vi "SFC_Get SOInfo.vi"(7 "UserNo":string, 8 "error in (no error)":errorcluster caption="错误输入（无错误）", 9 "Model":string, 10 "SalesOrder":string, 11 "Traceability 引用句柄":refnum<k24>) -> (0 "error out":errorcluster caption="错误输出", 2 ".NET:System.Data.DataSet":T1={"CaseSensitive"=FALSE, "Container"=refnum, "DataSetName"="", "DefaultViewManager"=refnum, "DesignMode"=FALSE, "EnforceConstraints"=FALSE, "ExtendedProperties"=refnum, "HasErrors"=FALSE, "IsInitialized"=FALSE, "Locale"=refnum, "Namespace"="", "Prefix"="", "Relations"=refnum, "RemotingFormat"=0, "SchemaSerializationMode"=1, "Site"=refnum, "Tables"=refnum} {"SchemaSerializationMode" items=["IncludeSchema"=1, "ExcludeSchema"=2]; "RemotingFormat" items=["Xml", "Binary"]}, 3 "Traceability 引用句柄输出":refnum<k24>)   [LabVIEW 2014, in "Traceability.lvlib"]
uses:
  D:/webservice/Traceability.dll
  Traceability.dll
  System.Data
  Traceability.lvlib
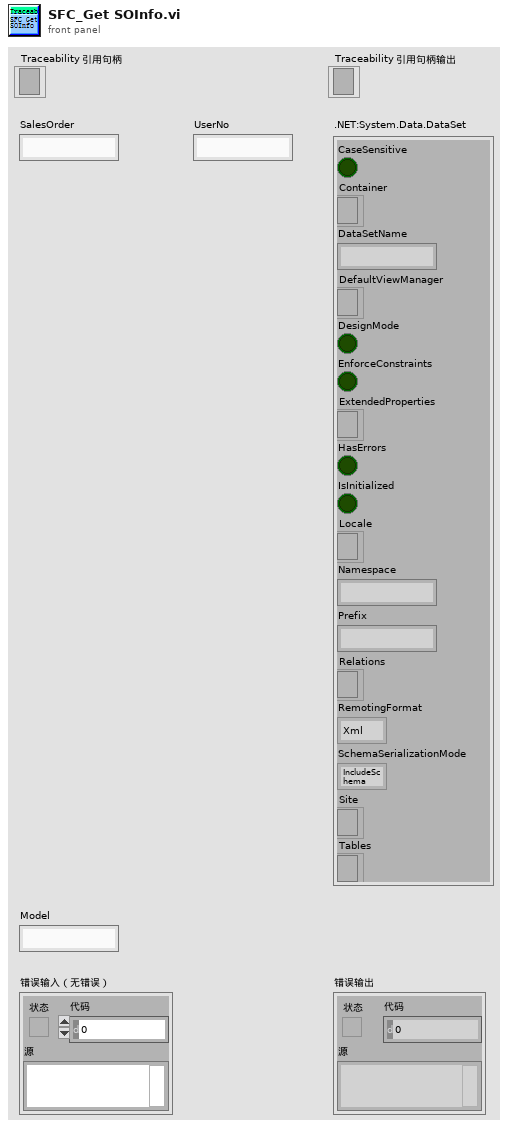
[diagram p1: front panel]
types:
  T1 = cluster{"CaseSensitive":bool, "Container":refnum<k24>, "DataSetName":string, "DefaultViewManager":refnum<k24>, "DesignMode":bool, "EnforceConstraints":bool, "ExtendedProperties":refnum<k24>, "HasErrors":bool, "IsInitialized":bool, "Locale":refnum<k24>, "Namespace":string, "Prefix":string, "Relations":refnum<k24>, "RemotingFormat":i32, "SchemaSerializationMode":i32, "Site":refnum<k24>, "Tables":refnum<k24>}
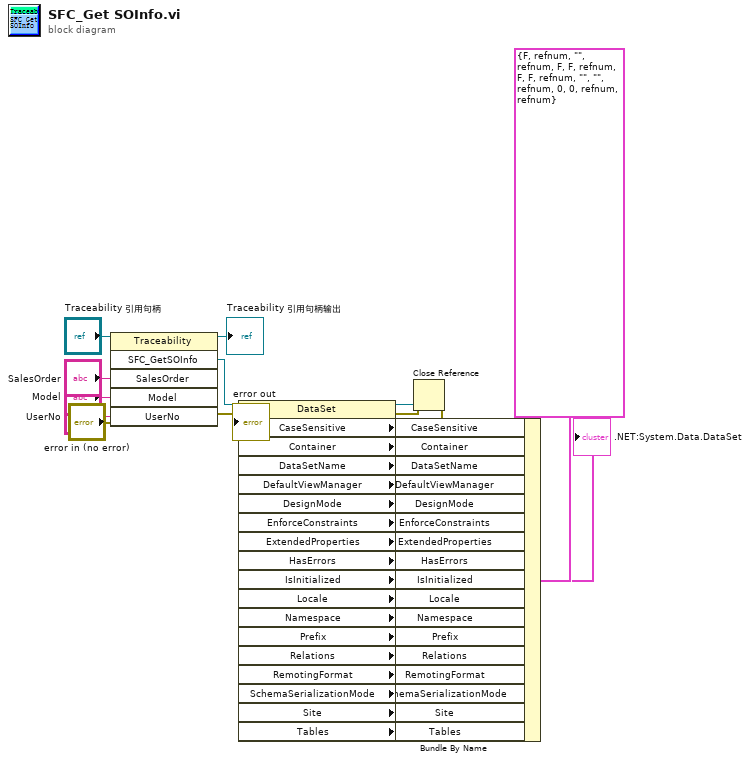
[diagram p0: block diagram]
diagram:
  n1 = invoke class="Traceability" method="SFC_GetSOInfo"(reference="Traceability 引用句柄", error in="error in (no error)", "SalesOrder"="SalesOrder", "Model"="Model", "UserNo"="UserNo") -> (reference out=→"Traceability 引用句柄输出":refnum<k24>, error out=w4:errorcluster, "SFC_GetSOInfo"=w27:refnum<k24>)  [unwired: 1 in, 3 out]
  n2 = property class="DataSet"(reference=w27, error in=w4) -> (reference out=w3:refnum<k24>, error out=w2:errorcluster, "CaseSensitive"=w24:bool, "Container"=w23:refnum<k24>, "DataSetName"=w22:string, "DefaultViewManager"=w21:refnum<k24>, "DesignMode"=w20:bool, "EnforceConstraints"=w19:bool, "ExtendedProperties"=w18:refnum<k24>, "HasErrors"=w17:bool, "IsInitialized"=w16:bool, "Locale"=w15:refnum<k24>, "Namespace"=w14:string, "Prefix"=w13:string, "Relations"=w12:refnum<k24>, "RemotingFormat"=w11:i32, "SchemaSerializationMode"=w10:i32, "Site"=w9:refnum<k24>, "Tables"=w8:refnum<k24>)
  n3 = Bundle By Name(cluster=T1 {"CaseSensitive"=FALSE, "Container"=refnum, "DataSetName"="", "DefaultViewManager"=refnum, "DesignMode"=FALSE, "EnforceConstraints"=FALSE, "ExtendedProperties"=refnum, "HasErrors"=FALSE, "IsInitialized"=FALSE, "Locale"=refnum, "Namespace"="", "Prefix"="", "Relations"=refnum, "RemotingFormat"=0, "SchemaSerializationMode"=0, "Site"=refnum, "Tables"=refnum} (".NET:System.Data.DataSet"), "CaseSensitive"=w24, "Container"=w23, "DataSetName"=w22, "DefaultViewManager"=w21, "DesignMode"=w20, "EnforceConstraints"=w19, "ExtendedProperties"=w18, "HasErrors"=w17, "IsInitialized"=w16, "Locale"=w15, "Namespace"=w14, "Prefix"=w13, "Relations"=w12, "RemotingFormat"=w11, "SchemaSerializationMode"=w10, "Site"=w9, "Tables"=w8) -> (→".NET:System.Data.DataSet":T1)
  n4 = Close Reference(reference=w3, error in (no error)=w2) -> (error out=→"error out":errorcluster)
